vi "getfractionalX_Bella.vi"(5 "CameraFlipped":T1=enum."on", 6 "screen [m]":dbl[](array[numeric]), 7 "start index (0)":i32, 9 "position [m]":dbl, 10 "pixelsize":dbl, 11 "position index":i32) -> (2 "index":dbl, 3 "position m":dbl)   [LabVIEW 2020]
uses:
  shared/OnOffTypeDef.ctl
panel:
  out "y value":dbl
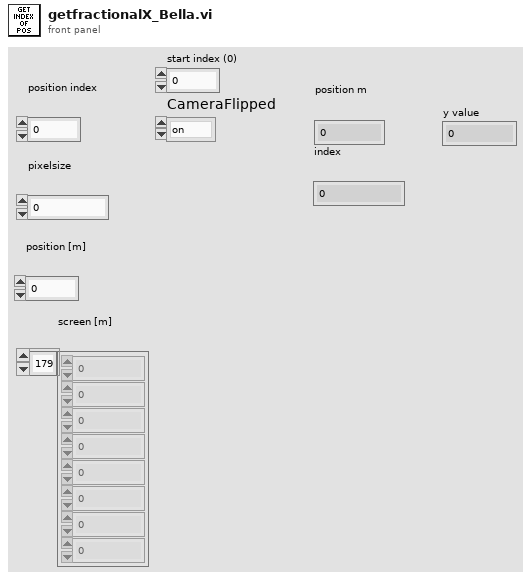
[diagram p1: front panel]
types:
  T1 = typedef "OnOffTypeDef.ctl" = enum16{"off", "on"}
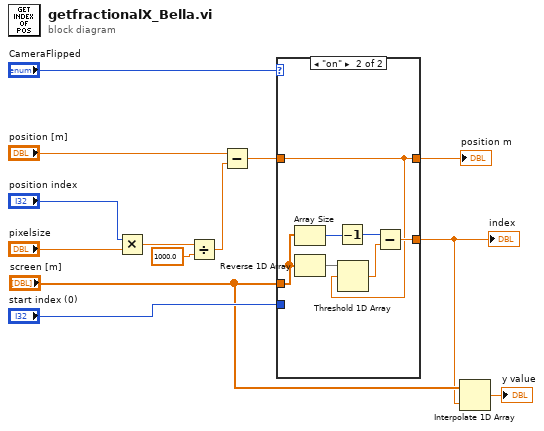
[diagram p0: block diagram]
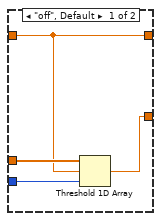
[diagram p2: hidden frame]
diagram:
  n1 = Multiply(x="position index", y="pixelsize") -> (x*y=w5:dbl)
  n2 = Divide(x=w5, y=1000.0) -> (x/y=w4:dbl)
  n3 = Subtract(x="position [m]", y=w4) -> (x-y=w3:dbl)
  n4 = case shown="\"on\"" "CameraFlipped" {
    tunnel: "screen [m]" -> [w17 w23]
    tunnel: w3 -> [w14 w18]
    tunnel: "start index (0)" -> [w16 _]
    tunnel: [w15 w21] -> w7
    tunnel: [w14 w18] -> w1
    frame "off", Default {
      n5 = Threshold 1D Array(1:w16, 2:w14, 3:w17) -> (0:w15:dbl)
    }
    frame "on" {
      n6 = Array Size(array=w23) -> (size(s)=w20:i32)
      n7 = Reverse 1D Array(array=w23) -> (reversed array=w24:dbl[])
      n8 = Decrement(x=w20) -> (x-1=w19:i32)
      n9 = Threshold 1D Array(2:w18, 3:w24) -> (0:w22:dbl)  [unwired: 1 in]
      n10 = Subtract(x=w19, y=w22) -> (x-y=w21:dbl)
    }
  }
  "position m" <- w1
  "index" <- w7
  n11 = Interpolate 1D Array(1:w7, 2:"screen [m]") -> (0:→"y value":dbl)
